vi "dfd_add () to Polynomial.vi"(4 "format control":T2={"Variable"="z", "Rendering Options"={"coefficients ascending order"=FALSE, "render ascending order"=TRUE, "negative exponent"=TRUE}}, 5 "fonts input":T5(array[cluster]), 6 "alignment(left, top)":T3, 7 "format string":string="%#.4g", 9 "rect in":T1, 10 "polynomial":dbl[](array[numeric]), 11 "picture in":picture) -> (1 "rect out":T1, 3 "new picture":picture)   [LabVIEW 2017, in "NI_DigFilter_Process.lvlib"]
uses:
  <vilib>/addons/Digital Filter Design/NI_DigFilter_Process.lvlib
  <vilib>/Analysis/polynomials.llb/Remove Zero Coefficients (DBL).vi
  <vilib>/Analysis/NI_AALPro.lvlib
panel:
  in  "desired font(user-specified font)":T4(ring)
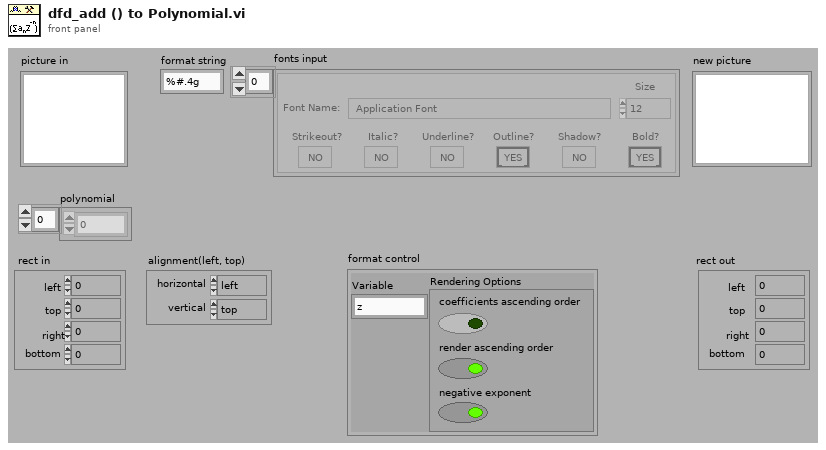
[diagram p1: front panel]
types:
  T1 = cluster{"left":i16, "top":i16, "right":i16, "bottom":i16}
  T2 = cluster{"Variable":string, "Rendering Options":cluster{"coefficients ascending order":bool, "render ascending order":bool, "negative exponent":bool}}
  T3 = cluster{"horizontal":enum16{"left", "center", "right"}, "vertical":enum16{"top", "center", "bottom"}}
  T4 = enum16{"User-specified Font", "Application Font", "System Font", "Dialog Font"}
  T5 = cluster{"Font Name:":string, "Size":i16, "Strikeout?":bool, "Italic?":bool, "Underline?":bool, "Outline?":bool, "Shadow?":bool, "Bold?":bool}[]
  T6 = cluster{"Font Name:":string, "Size":i16, "Strikeout?":bool, "Italic?":bool, "Underline?":bool, "Outline?":bool, "Shadow?":bool, "Bold?":bool}
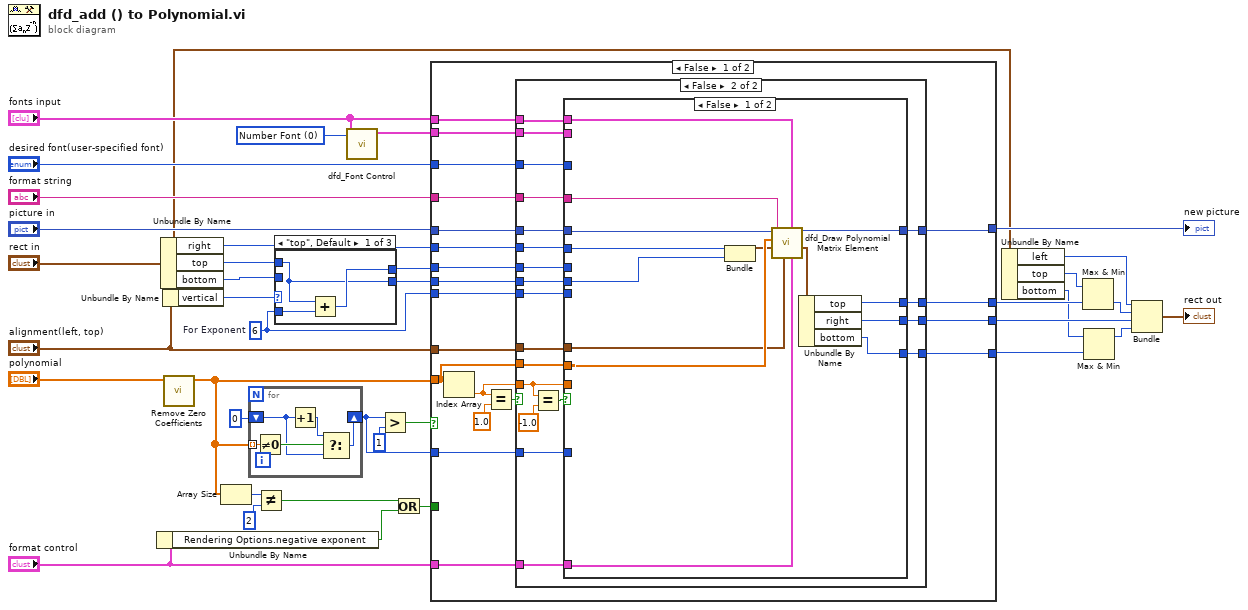
[diagram p0: block diagram]
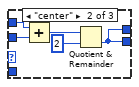
[diagram p2: hidden frame]
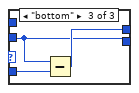
[diagram p3: hidden frame]
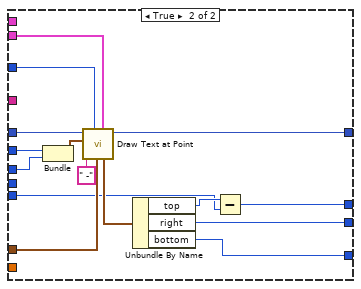
[diagram p5: hidden frame]
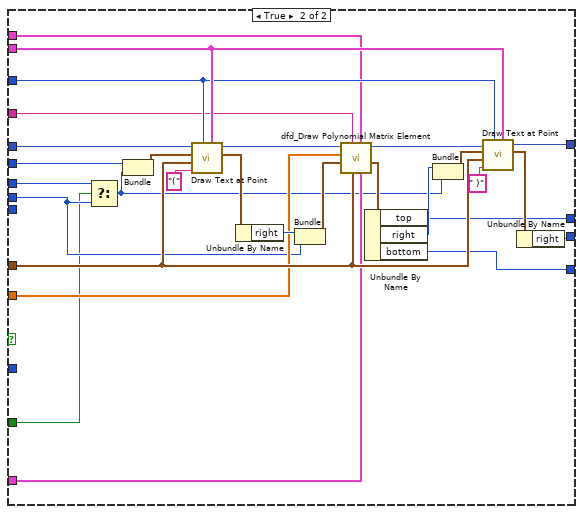
[diagram p6: hidden frame]
diagram:
  w25 = u16 0 items=["Number Font", "Variable Font", "Script Font"] ("Tpye")
  w19 = 6  # For Exponent
  n1 = Unbundle By Name("format control") -> ("Rendering Options.negative exponent"=w2:bool)
  n2 = Unbundle By Name("rect in") -> ("right"=w28:i16, "top"=w18:i16, "bottom"=w16:i16)
  n3 = Unbundle By Name("alignment(left, top)") -> ("vertical"=w26:enum16{"top", "center", "bottom"})
  n4 = call-poly <vilib>:"Remove Zero Coefficients.vi"("P(x) In"="polynomial") -> ("P(x) Out"=w3:dbl[])  [unwired: 2 in, 8 out]
  n5 = Array Size(array=w3) -> (size(s)=w4:i32)
  n6 = for {
    shift-right: [w38] -> w20
    shift-left: 0 -> [w40]
    tunnel: w3 -> [w42] mode=indexing
    n7 = Not Equal To 0?(x=w42) -> (x != 0?=w41:bool)
    n8 = Increment(x=w40) -> (x+1=w39:i32)
    n9 = Select(t=w39, s=w41, f=w40) -> (s? t:f=w38:i32)
  }
  n10 = Not Equal?(x=w4, y=2) -> (x != y?=w6:bool)
  n11 = case shown="\"top\", Default" w26 {
    tunnel: w18 -> [w44 w50 _]
    tunnel: [w45 w46 w52] -> w22
    tunnel: [w44 w46 w51] -> w21
    tunnel: w19 -> [w43 _ w53]
    tunnel: w16 -> [_ w49 w51]
    frame "top", Default {
      n12 = Add(x=w44, y=w43) -> (x+y=w45:i32)
    }
    frame "center" {
      n13 = Add(x=w50, y=w49) -> (x+y=w48:i16)
      n14 = Quotient & Remainder(x=w48, y=i16 2) -> (floor(x/y)=w46:i16)  [unwired: 1 out]
    }
    frame "bottom" {
      n15 = Subtract(x=w51, y=w53) -> (x-y=w52:i32)
    }
  }
  n16 = call <vilib>:"dfd_Font Control.vi"("tpye"=w25, "fonts input"="fonts input") -> ("font output"=w23:T6)  [unwired: 9 out]
  n17 = Greater?(x=w20, y=1) -> (0:w35:bool)
  n18 = Or(x=w6, y=w2) -> (x .or. y?=w1:bool)
  n19 = case shown="False" w35 {
    tunnel: "desired font(user-specified font)" -> [w70 w141]
    tunnel: "fonts input" -> [w64 w139]
    tunnel: w3 -> [w66 w130]
    tunnel: "picture in" -> [w68 w147]
    tunnel: w28 -> [w63 w151]
    tunnel: w22 -> [w67 w129]
    tunnel: w21 -> [w61 w128]
    tunnel: [w62 w145] -> w30
    tunnel: "format string" -> [w69 w138]
    tunnel: [w60 w150] -> w29
    tunnel: w23 -> [w71 w142]
    tunnel: "alignment(left, top)" -> [w59 w134]
    tunnel: [w58 w133] -> w11
    tunnel: w19 -> [w57 _]
    tunnel: w20 -> [w56 _]
    tunnel: "format control" -> [w55 w131]
    tunnel: [w54 w132] -> w9
    tunnel: w1 -> [_ w126]
    frame False {
      n20 = Index Array(array=w66) -> (element=w65:dbl)  [unwired: 1 in]
      n21 = Equal?(x=w65, y=1.0) -> (x = y?=w72:bool)
      n22 = case shown="False" w72 {
        tunnel: w71 -> [_ w96]
        tunnel: w70 -> [_ w95]
        tunnel: w69 -> [_ w94]
        tunnel: w68 -> [w76 w93]
        tunnel: w67 -> [_ w84]
        tunnel: w66 -> [_ w92]
        tunnel: w65 -> [_ w80]
        tunnel: w64 -> [_ w89]
        tunnel: w63 -> [w75 w88]
        tunnel: [w76 w87] -> w62
        tunnel: [w75 w86] -> w60
        tunnel: w61 -> [w74 w85]
        tunnel: w59 -> [_ w83]
        tunnel: [w74 w82] -> w58
        tunnel: w57 -> [_ w81]
        tunnel: w56 -> [_ w79]
        tunnel: w55 -> [_ w78]
        tunnel: [w74 w77] -> w54
        frame True {
        }
        frame False {
          n23 = Equal?(x=w80, y=-1.0) -> (x = y?=w90:bool)
          n24 = case shown="False" w90 {
            tunnel: w93 -> [w107 w123]
            tunnel: w95 -> [_ w122]
            tunnel: w88 -> [w109 w121]
            tunnel: w85 -> [w97 _]
            tunnel: [w106 w119] -> w87
            tunnel: [w110 w118] -> w86
            tunnel: w96 -> [_ w117]
            tunnel: w94 -> [w104 _]
            tunnel: w92 -> [w103 _]
            tunnel: w89 -> [w105 _]
            tunnel: w84 -> [_ w116]
            tunnel: w83 -> [w102 w115]
            tunnel: [w108 w113] -> w82
            tunnel: w81 -> [_ w112]
            tunnel: w80 -> [_ _]
            tunnel: w79 -> [_ _]
            tunnel: w78 -> [w99 _]
            tunnel: [w98 w111] -> w77
            frame False {
              n25 = Bundle("right"=w109, "bottom"=w97) -> (w100:cluster{"right":i16, "bottom":i16})  [unwired: 1 out]
              n26 = call <vilib>:"dfd_Draw Polynomial Matrix Element.vi"("format control"=w99, "fonts input"=w105, "alignment(left, top)"=w102, "format string"=w104, "origin"=w100, "coefficients"=w103, "picture in"=w107) -> ("location"=w101:T1, "picture out"=w106:picture)  [unwired: 3 out]
              n27 = Unbundle By Name(w101) -> ("top"=w108:i16, "right"=w110:i16, "bottom"=w98:i16)
            }
            frame True {
              n28 = Bundle("right"=w121, w116) -> (w120:cluster{"right":i16, i32})  [unwired: 1 out]
              n29 = call <vilib>:"Draw Text at Point.vi"("[user-specified font]"=w117, "desired font(Application)"=w122, "text"=" -", "alignment(left, top)"=w115, "origin"=w120, "picture"=w123) -> ("text rect"=w124:T1, "new picture"=w119:picture)  [unwired: 3 in, 1 out]
              n30 = Unbundle By Name(w124) -> ("top"=w114:i16, "right"=w118:i16, "bottom"=w111:i16)
              n31 = Subtract(x=w114, y=w112) -> (x-y=w113:i32)
            }
          }
        }
      }
    }
    frame True {
      n32 = Select(t=w129, s=w126, f=w128) -> (s? t:f=w127:i32)
      n33 = Bundle("right"=w151, "bottom"=w127) -> (w149:cluster{"right":i16, "bottom":i32})  [unwired: 1 out]
      n34 = call <vilib>:"Draw Text at Point.vi"("[user-specified font]"=w142, "desired font(Application)"=w141, "text"="(", "alignment(left, top)"=w134, "origin"=w149, "picture"=w147) -> ("text rect"=w154:T1, "new picture"=w140:picture)  [unwired: 3 in, 1 out]
      n35 = Unbundle By Name(w154) -> ("right"=w153:i16)
      n36 = Bundle("right"=w153, "bottom"=w128) -> (w135:cluster{"right":i16, "bottom":i16})  [unwired: 1 out]
      n37 = call <vilib>:"dfd_Draw Polynomial Matrix Element.vi"("format control"=w131, "fonts input"=w139, "alignment(left, top)"=w134, "format string"=w138, "origin"=w135, "coefficients"=w130, "picture in"=w140) -> ("location"=w136:T1, "picture out"=w137:picture)  [unwired: 3 out]
      n38 = Unbundle By Name(w136) -> ("top"=w133:i16, "right"=w152:i16, "bottom"=w132:i16)
      n39 = Bundle("right"=w152, "bottom"=w127) -> (w143:cluster{"right":i16, "bottom":i32})  [unwired: 1 out]
      n40 = call <vilib>:"Draw Text at Point.vi"("[user-specified font]"=w142, "desired font(Application)"=w141, "text"=" )", "alignment(left, top)"=w134, "origin"=w143, "picture"=w137) -> ("text rect"=w144:T1, "new picture"=w145:picture)  [unwired: 3 in, 1 out]
      n41 = Unbundle By Name(w144) -> ("right"=w150:i16)
    }
  }
  "new picture" <- w30
  n42 = Unbundle By Name("rect in") -> ("left"=w14:i16, "top"=w13:i16, "bottom"=w10:i16)
  n43 = Max & Min(x=w13, y=w11) -> (min(x,y)=w17:i32)  [unwired: 1 out]
  n44 = Max & Min(x=w10, y=w9) -> (max(x,y)=w12:i16)  [unwired: 1 out]
  n45 = Bundle("left"=w14, w17, "right"=w29, w12) -> (→"rect out":cluster{"left":i16, i32, "right":i16, i16})  [unwired: 1 out]
